vi "CarWashServerData(subVI).vi"(8 "error in (no error)":errorcluster) -> (0 "error out":errorcluster, 2 "Wash Data":string[][](table), 3 "Wash Data in Wave Form":i32[][](graph))   [LabVIEW 2024]
uses:
  <vilib>/Utility/file.llb/Read Delimited Spreadsheet (string).vi
  <vilib>/Utility/file.llb/Write Delimited Spreadsheet (string).vi
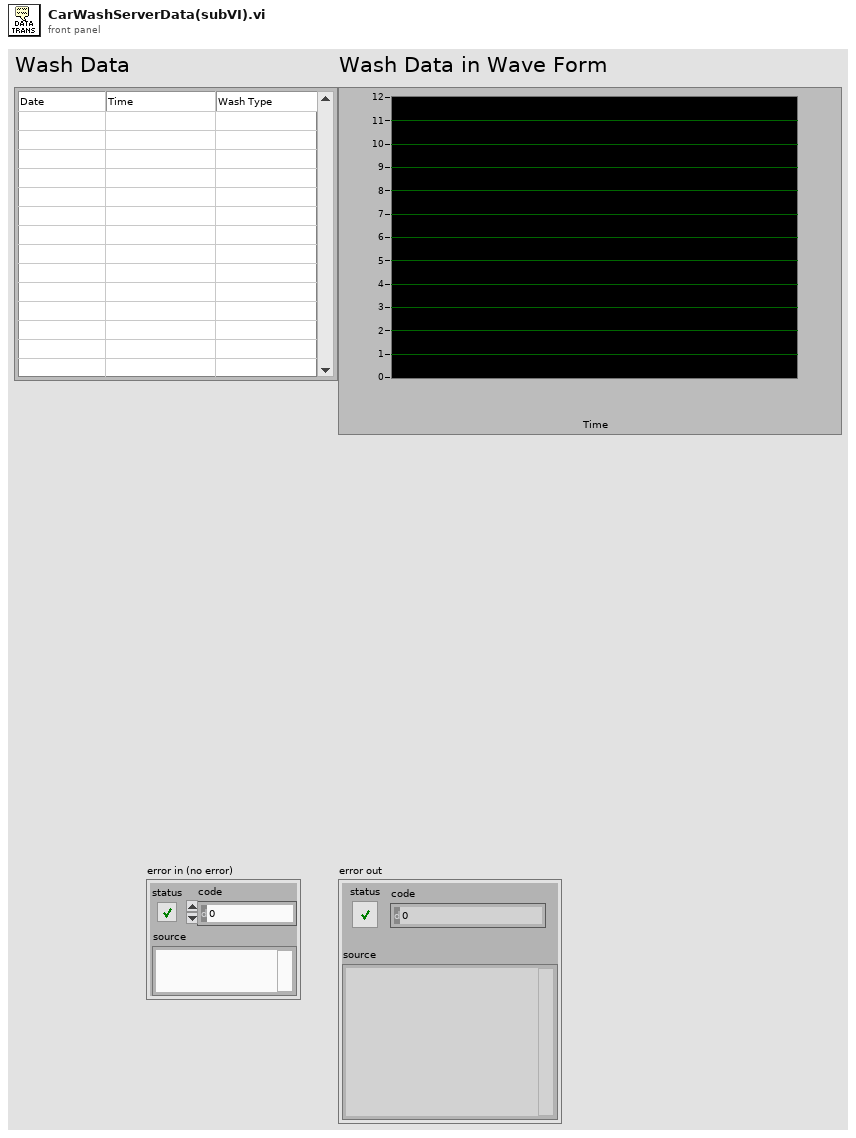
[diagram p1: front panel]
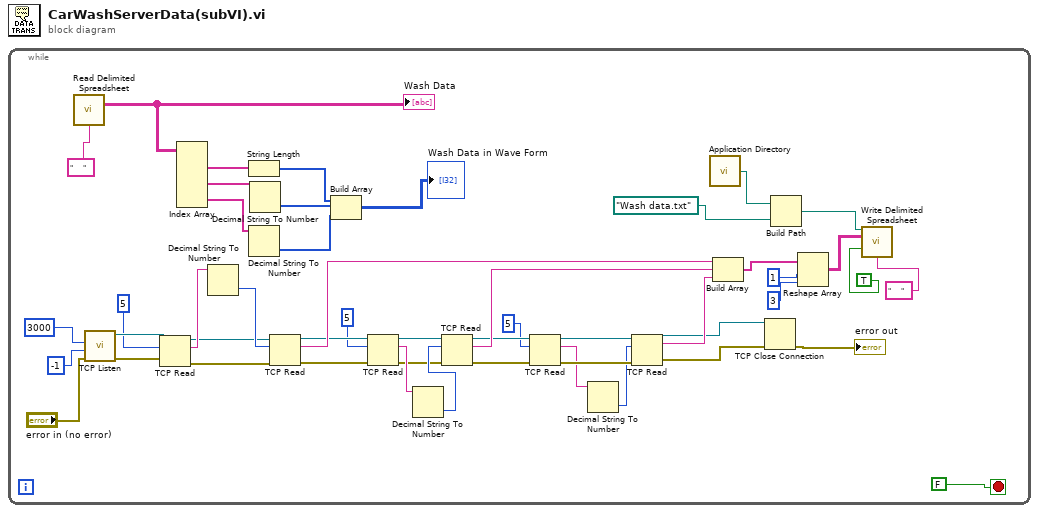
[diagram p0: block diagram]
diagram:
  n1 = while {
    stop <- FALSE stop-if-true
    n2 = call-poly <vilib>:"Read Delimited Spreadsheet.vi"("delimiter (\\t)"="     " ("delimiter (\\t)")) -> ("all rows"=w10:string[][])  [unwired: 9 in, 5 out]
    "Wash Data" <- w10
    n3 = call <vilib>:"TCP Listen.vi"("error in (no error)"="error in (no error)", "timeout ms (wait forever: -1)"=-1, "port"=u16 3000) -> ("error out"=w27:errorcluster, "connection ID"=w26:refnum<k5>)  [unwired: 4 in, 3 out]
    n4 = TCP Read(connection ID=w26, bytes to read=5, error in (no error)=w27) -> (connection ID out=w28:refnum<k5>, data out=w40:string, error out=w29:errorcluster)  [unwired: 2 in]
    n5 = Index Array(array=w10) -> (element #1=w9:string[], element #2=w8:string[], element #3=w7:string[])  [unwired: 6 in]
    n6 = Decimal String To Number(string=w40) -> (number=w41:i32)  [unwired: 2 in, 1 out]
    n7 = String Length(string=w9) -> (length=w6:i32[])
    n8 = Decimal String To Number(string=w7) -> (number=w4:i32[])  [unwired: 2 in, 1 out]
    n9 = Decimal String To Number(string=w8) -> (number=w5:i32[])  [unwired: 2 in, 1 out]
    n10 = TCP Read(connection ID=w28, bytes to read=w41, error in (no error)=w29) -> (connection ID out=w30:refnum<k5>, data out=w47:string, error out=w31:errorcluster)  [unwired: 2 in]
    n11 = Build Array(w6, w5, w4) -> (→"Wash Data in Wave Form":i32[][])
    n12 = TCP Read(connection ID=w30, bytes to read=5, error in (no error)=w31) -> (connection ID out=w32:refnum<k5>, data out=w42:string, error out=w33:errorcluster)  [unwired: 2 in]
    n13 = Decimal String To Number(string=w42) -> (number=w43:i32)  [unwired: 2 in, 1 out]
    n14 = TCP Read(connection ID=w32, bytes to read=w43, error in (no error)=w33) -> (connection ID out=w34:refnum<k5>, data out=w46:string, error out=w35:errorcluster)  [unwired: 2 in]
    n15 = TCP Read(connection ID=w34, bytes to read=5, error in (no error)=w35) -> (connection ID out=w36:refnum<k5>, data out=w15:string, error out=w37:errorcluster)  [unwired: 2 in]
    n16 = Decimal String To Number(string=w15) -> (number=w14:i32)  [unwired: 2 in, 1 out]
    n17 = TCP Read(connection ID=w36, bytes to read=w14, error in (no error)=w37) -> (connection ID out=w38:refnum<k5>, data out=w45:string, error out=w39:errorcluster)  [unwired: 2 in]
    n18 = call <vilib>:"Application Directory.vi"() -> ("Application Directory"=w2:path)
    n19 = Build Array "Build Array"(w47, w46, w45) -> (w20:string[])
    n20 = TCP Close Connection(connection ID=w38, error in (no error)=w39) -> (error out=→"error out":errorcluster)  [unwired: 1 in, 1 out]
    n21 = Build Path(base path=w2, name or relative path=path "Wash data.txt") -> (appended path=w48:path)
    n22 = Reshape Array(w20, 1 ("dimension size"), 3 ("dimension size")) -> (w17:string[][])
    n23 = call-poly <vilib>:"Write Delimited Spreadsheet.vi"("file path (dialog if empty)"=w48, "2D data"=w17, "append to file? (new file:F)"=TRUE, "delimiter (\\t)"="     " ("delimiter (\\t)")) -> ()  [unwired: 10 in, 2 out]
  }
